vi "File Viewer v5.vi"() -> ()   [LabVIEW 2019]
uses:
  <vilib>/Utility/file.llb/Read Delimited Spreadsheet (I64).vi
  <vilib>/Utility/file.llb/Write Delimited Spreadsheet (DBL).vi
panel:
  in  "Stop":bool
  in  "Tab Control":T1(tab)
  in  "IR Filter:":u16(ring) items=["No filter", "100 nm Al", "200 nm Al", "250 nm Al", "500 nm Al"]
  in  "update":bool
  out "Raw Image From Camera":i32[][](graph)
  in  "File Path for Image:":path
  out "Expected position on spectrometer (pixels):":dbl
  in  "Grating:":u16(ring) items=["Shimadzu 30-006  "]
  in  "Laser:":u16(ring) items=["800nm  "]
  in  "Harmonic":dbl min=10.0 max=40.0
  out "l (nm)":dbl
  out "E (J)":dbl
  out "E (eV)":dbl
  out "Nearest Harmonic of 800nm":dbl
  out "Vertical Binned Waveform Graph":i64[](graph)
  out "Cursor Position (pixels)":dbl
  out "Distance to nearest harmonic of 800nm (pixels)":dbl
  in  "Caibration Date":u16(ring) items=["first calibration - 7/31", "7/31-current"]
  in  "Correct for QE?":bool
  in  "Save text file":bool
  in  "Graph to export:":u16(ring) items=["Wavelength Graph", "Energy Graph", "Harmonics Graph"]
  out "Wavelength Graph":T2(graph)
  out "Energy Graph (eV)":cluster{"eV":dbl, "QE scaled count":dbl}[](graph)
  out "Harmonics Graph":cluster{dbl, "QE scaled count":dbl}[](graph)
  in  "Pump/Probe Run Folder:":path
  out "Distance to nearest harmonic of 800nm (pixels)":dbl
  out "Cursor Position on CCD  (pixels)":dbl
  out "Nearest Harmonic of 800nm":dbl
  out "E (eV) 2":dbl
  out "E (J)":dbl
  out "l (nm)":dbl
  in  "Pump/Probe Harmonic:":dbl min=10.0 max=40.0
  out "Expected position on spectrometer (pixels):":dbl
  out "Time delay":dbl
  out "XUV":dbl[][](graph)
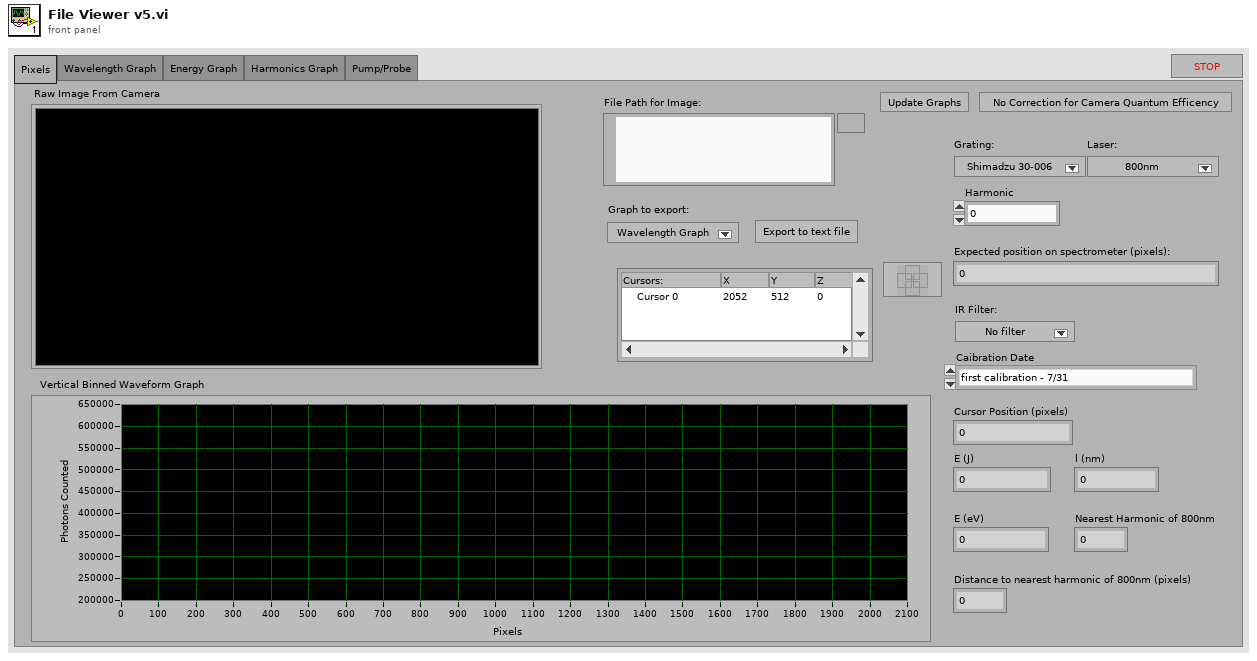
[diagram p1: front panel]
types:
  T1 = enum32{"Pixels", "Wavelength Graph", "Energy Graph", "Harmonics Graph", "Pump/Probe"}
  T2 = cluster{"No prefix":dbl, "QE scaled count":dbl}[]
  T3 = cluster{"No prefix":dbl, "filter scaled count":dbl}
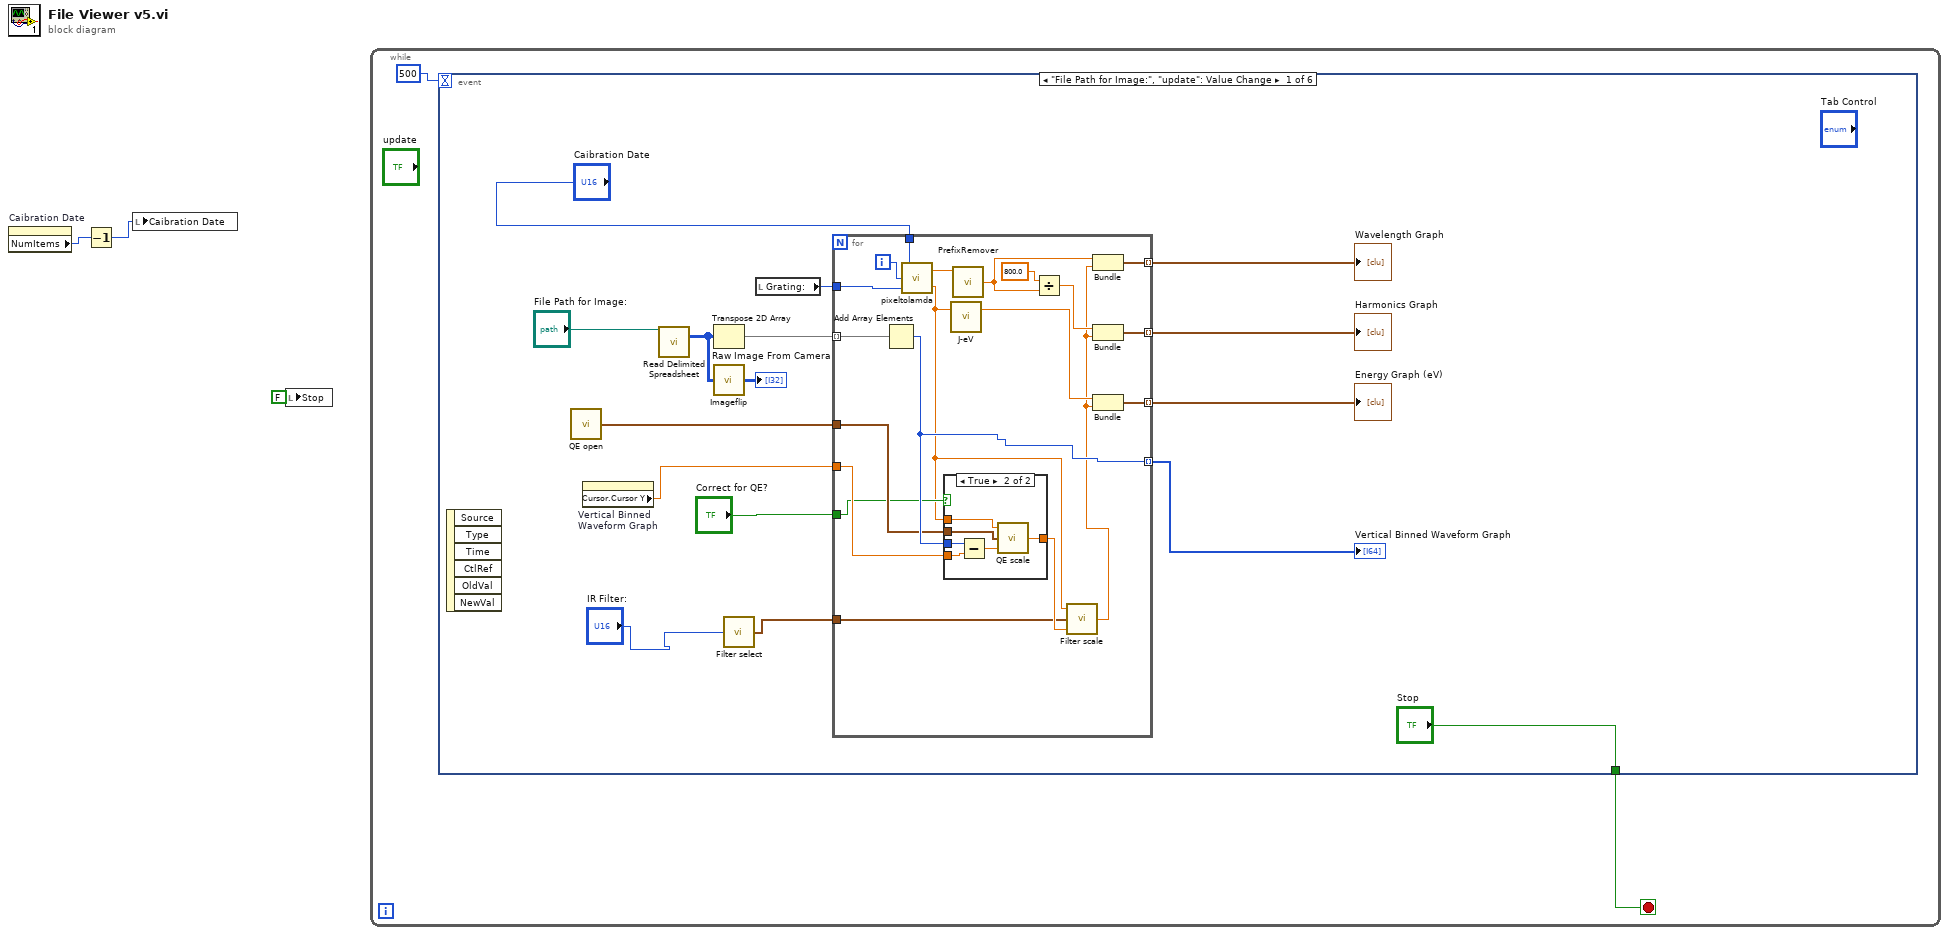
[diagram p0: block diagram]
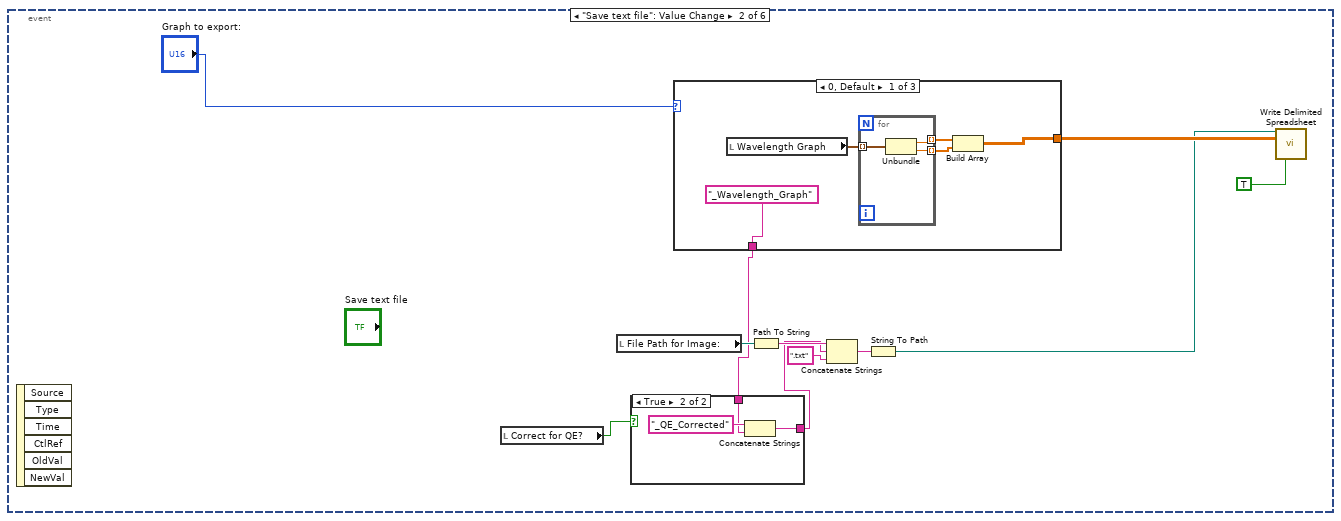
[diagram p3: hidden frame]
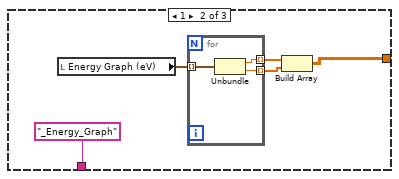
[diagram p5: hidden frame]
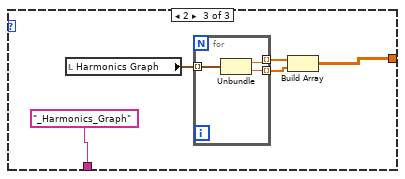
[diagram p6: hidden frame]
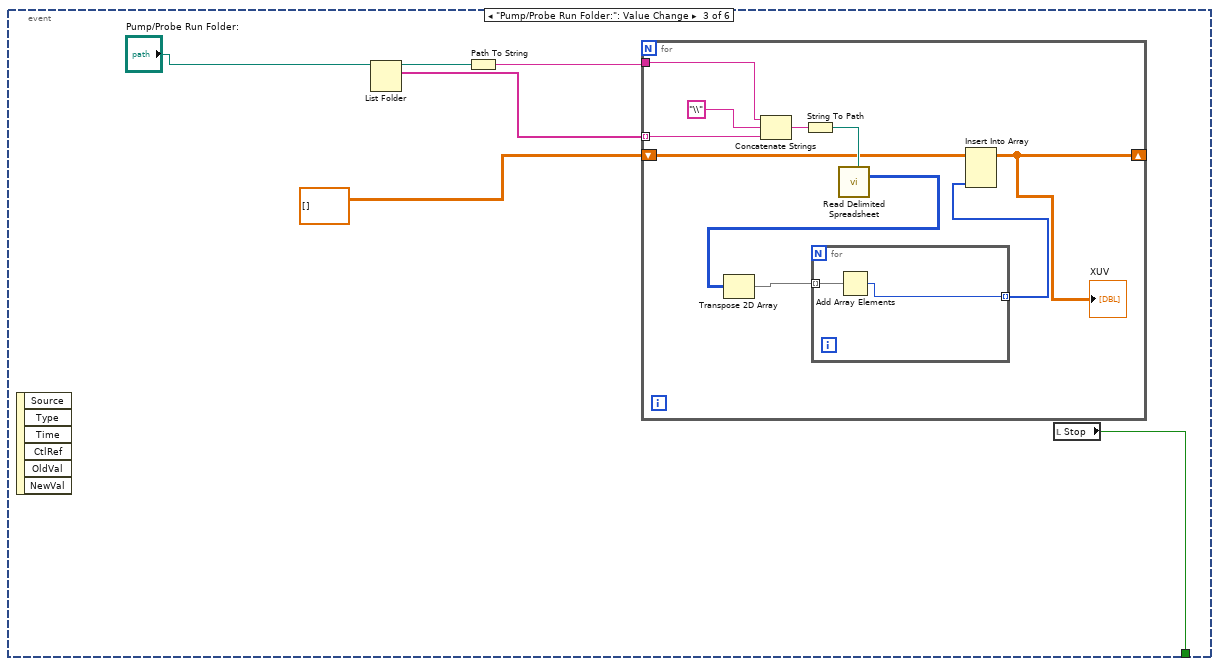
[diagram p7: hidden frame]
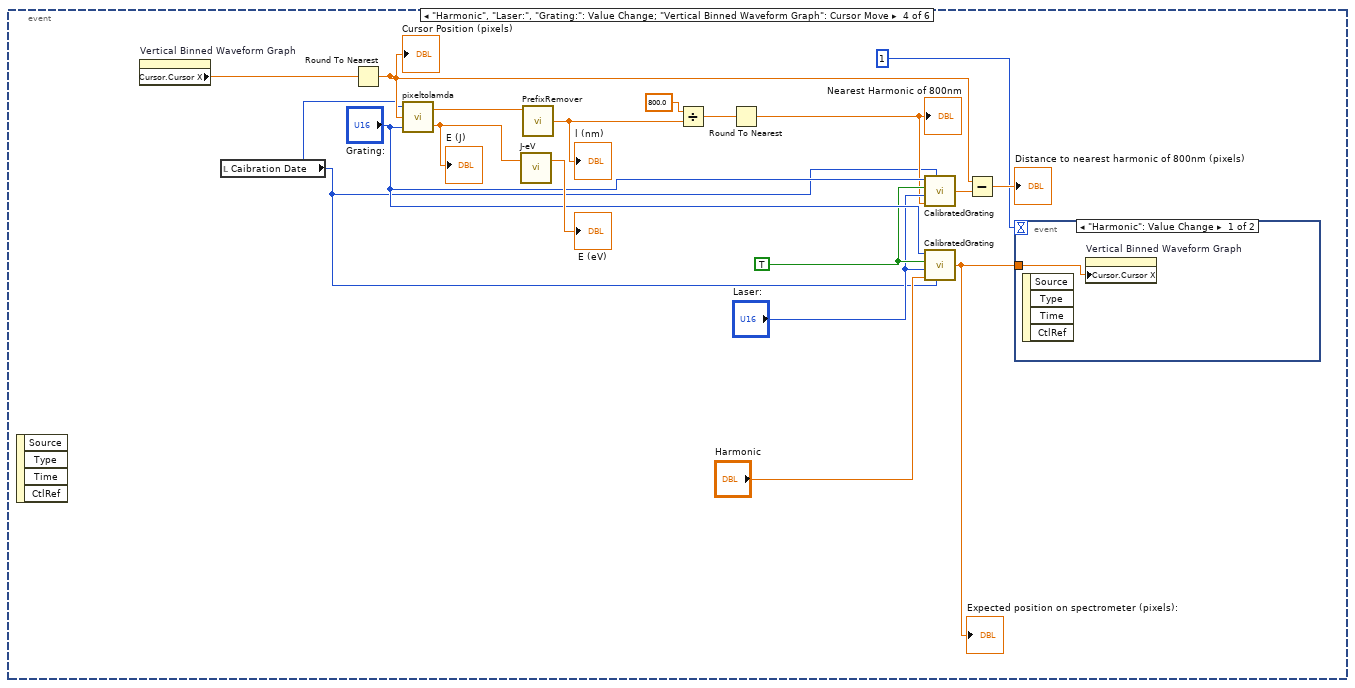
[diagram p8: hidden frame]
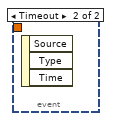
[diagram p9: hidden frame]
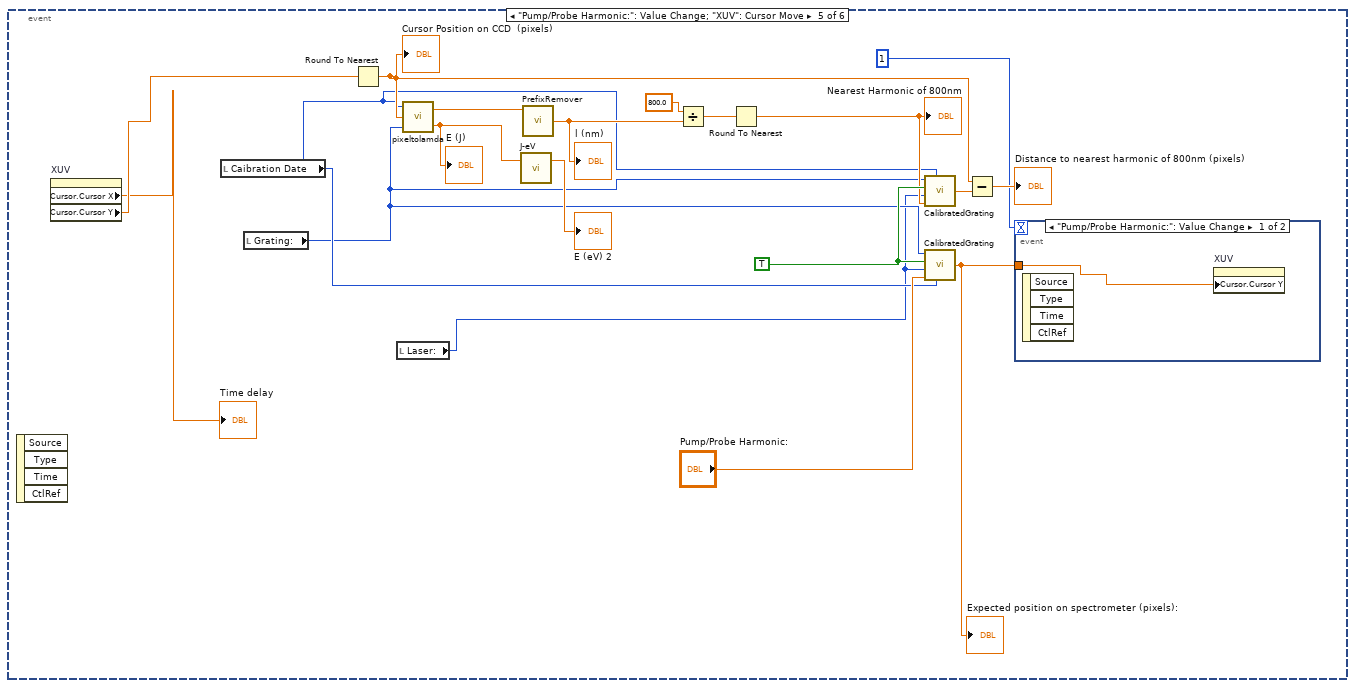
[diagram p10: hidden frame]
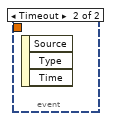
[diagram p11: hidden frame]
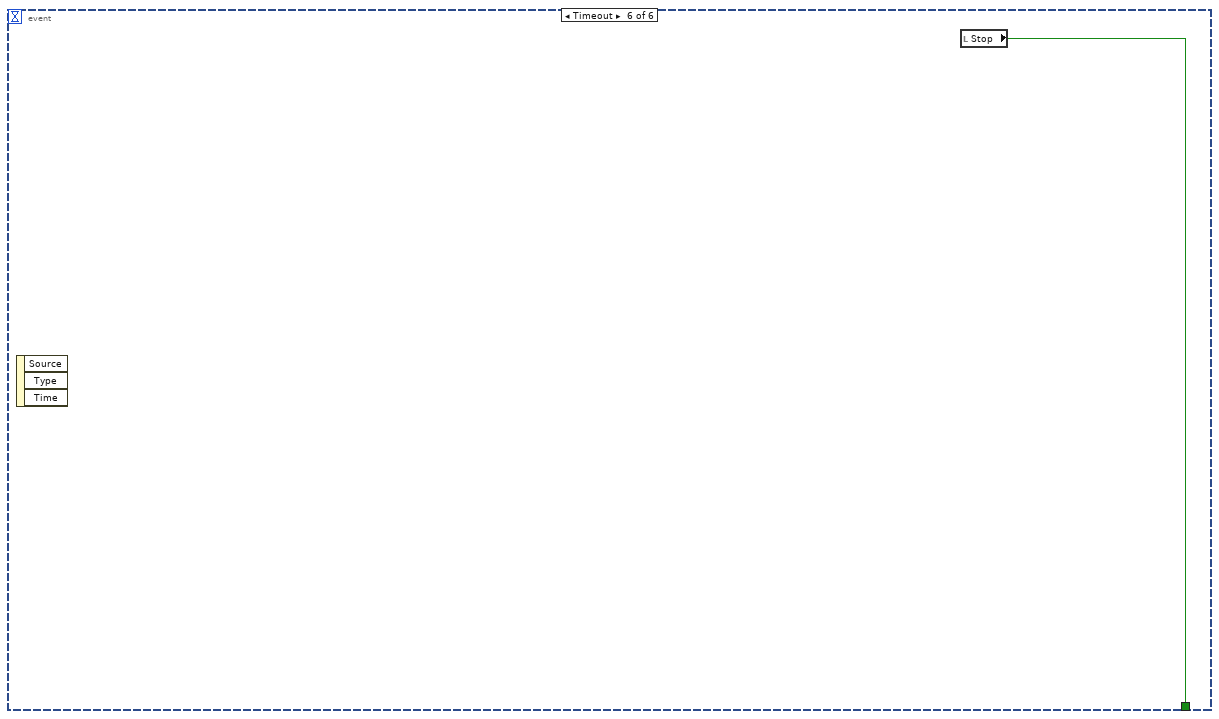
[diagram p12: hidden frame]
diagram:
  n1 = property on="Caibration Date" class="Ring (strict)"() -> ("NumItems"=w1:u32)  [unwired: 2 in, 2 out]
  n2 = Decrement(x=w1) -> (x-1=w2:u32)
  n3 = local write "Caibration Date"(w2) -> ()
  n4 = local write "Stop"(FALSE) -> ()
  n5 = while {
    stop <- w5 stop-if-true
    n6 = event shown="[0] \"File Path for Image:\", \"update\": Value Change" {
      selector: _ -> [_ _ _ _ _ _]
      dyn-events: _ -> [_ _ _ _ _ _]
      timeout: 500 -> [_ _ _ _ _ _]
      tunnel: ["Stop" _ w89 _ _ w145] -> w5
      event "File Path for Image:", "update": Value Change {
        n7 = event-data() -> ()  [unwired: 1 in, 6 out]
        n8 = call "QE open.vi"() -> ("QE data"=w10:cluster{"Numeric":dbl, dbl}[])
        n9 = property on="Vertical Binned Waveform Graph" class="WFGraph (strict)"() -> ("Cursor.Cursor Y"=w9:dbl)  [unwired: 2 in, 2 out]
        n10 = call-poly <vilib>:"Read Delimited Spreadsheet.vi"("file path (dialog if empty)"="File Path for Image:") -> ("all rows"=w18:i64[][])  [unwired: 9 in, 5 out]
        n11 = Transpose 2D Array(2D array=w18) -> (transposed array=w17:i64[][])
        n12 = call "Imageflip.vi"("2D array"=w18) -> ("transposed array"=→"Raw Image From Camera":i32[][])
        n13 = call "Filter select.vi"("Filter:"="IR Filter:") -> ("filter data"=w6:cluster{"Numeric":dbl, dbl}[])
        n14 = local read "Grating:"() -> (w15:u16)
        n15 = for {
          tunnel: w17 -> [w41] mode=indexing
          tunnel: [w29] -> w16 mode=indexing
          tunnel: w15 -> [w39]
          tunnel: [w38] -> w14 mode=indexing
          tunnel: [w37] -> w13 mode=indexing
          tunnel: [w32] -> w12 mode=indexing
          tunnel: "Caibration Date" -> [w31]
          tunnel: w10 -> [w28]
          tunnel: w9 -> [w30]
          tunnel: "Correct for QE?" -> [w26]
          tunnel: w6 -> [w22]
          i -> [w40]
          n16 = Add Array Elements(numeric array=w41) -> (sum=w29:i64)
          n17 = call "pixeltolamda.vi"("Grating:"=w39, "Pixel Postion"=w40, "Caibration Date"=w31) -> ("E (J)"=w23:dbl, "lamda (m)"=w35:dbl)
          n18 = case shown="True" w26 {
            tunnel: w30 -> [_ w48]
            tunnel: w29 -> [w42 w47]
            tunnel: w28 -> [_ w44]
            tunnel: w23 -> [_ w45]
            tunnel: [w42 w46] -> w25
            frame False {
            }
            frame True {
              n19 = Subtract(x=w47, y=w48) -> (x-y=w43:dbl)
              n20 = call "QE scale.vi"("Raw Photon Count"=w43, "QE data"=w44, "Energy (J)"=w45) -> ("QE scaled count"=w46:dbl)
            }
          }
          n21 = call "J-eV.vi"("J"=w23) -> ("eV"=w27:dbl)  [unwired: 1 in, 1 out]
          n22 = call "PrefixRemover.vi"("Nano"=w35) -> ("No prefix"=w34:dbl)  [unwired: 3 in]
          n23 = Divide(x=800.0, y=w34) -> (x/y=w33:dbl)
          n24 = call "Filter scale.vi"("Raw Photon Count"=w25, "filter data"=w22, "Energy (J)"=w23) -> ("filter scaled count"=w24:dbl)
          n25 = Bundle("No prefix"=w34, "filter scaled count"=w24) -> (w38:T3)  [unwired: 1 in]
          n26 = Bundle(w33, "filter scaled count"=w24) -> (w32:cluster{dbl, "filter scaled count":dbl})  [unwired: 1 in]
          n27 = Bundle("eV"=w27, "filter scaled count"=w24) -> (w37:cluster{"eV":dbl, "filter scaled count":dbl})  [unwired: 1 in]
        }
        "Vertical Binned Waveform Graph" <- w16
        "Wavelength Graph" <- w14
        "Energy Graph (eV)" <- w13
        "Harmonics Graph" <- w12
      }
      event "Save text file": Value Change {
        n28 = event-data() -> ()  [unwired: 1 in, 6 out]
        n29 = local read "Correct for QE?"() -> (w53:bool)
        n30 = local read "File Path for Image:"() -> (w56:path)
        n31 = case shown="0, Default" "Graph to export:" {
          tunnel: [w65 w73 w81] -> w58
          tunnel: ["_Wavelength_Graph" ("pattern (all files)") "_Energy_Graph" ("pattern (all files)") "_Harmonics_Graph" ("pattern (all files)")] -> w51
          frame 0, Default {
            n32 = local read "Wavelength Graph"() -> (w68:T2)
            n33 = for {
              tunnel: w68 -> [w71] mode=indexing
              tunnel: [w70] -> w67 mode=indexing
              tunnel: [w69] -> w66 mode=indexing
              n34 = Unbundle(w71) -> ("No prefix"=w70:dbl, "QE scaled count"=w69:dbl)
            }
            n35 = Build Array(w67, w66) -> (w65:dbl[][])
          }
          frame 1 {
            n36 = local read "Energy Graph (eV)"() -> (w74:cluster{"eV":dbl, "QE scaled count":dbl}[])
            n37 = for {
              tunnel: w74 -> [w79] mode=indexing
              tunnel: [w78] -> w76 mode=indexing
              tunnel: [w77] -> w75 mode=indexing
              n38 = Unbundle(w79) -> ("eV"=w78:dbl, "QE scaled count"=w77:dbl)
            }
            n39 = Build Array(w76, w75) -> (w73:dbl[][])
          }
          frame 2 {
            n40 = local read "Harmonics Graph"() -> (w82:cluster{dbl, "QE scaled count":dbl}[])
            n41 = for {
              tunnel: w82 -> [w87] mode=indexing
              tunnel: [w86] -> w84 mode=indexing
              tunnel: [w85] -> w83 mode=indexing
              n42 = Unbundle(w87) -> (w86:dbl, "QE scaled count"=w85:dbl)
            }
            n43 = Build Array(w84, w83) -> (w81:dbl[][])
          }
        }
        n44 = case shown="True" w53 {
          tunnel: [w60 w62] -> w52
          tunnel: w51 -> [w60 w61]
          frame False {
          }
          frame True {
            n45 = Concatenate Strings("_QE_Corrected" ("pattern (all files)"), w61) -> (w62:string)
          }
        }
        n46 = Path To String(path=w56) -> (string=w55:string)
        n47 = Concatenate Strings(w55, w52, ".txt" ("pattern (all files)")) -> (w50:string)
        n48 = String To Path(string=w50) -> (path=w49:path)
        n49 = call-poly <vilib>:"Write Delimited Spreadsheet.vi"("file path (dialog if empty)"=w49, "2D data"=w58, "transpose? (no:F)"=TRUE) -> ()  [unwired: 11 in, 2 out]
      }
      event "Pump/Probe Run Folder:": Value Change {
        n50 = event-data() -> ()  [unwired: 1 in, 6 out]
        n51 = List Folder(path="Pump/Probe Run Folder:") -> (path out=w91:path, filenames=w92:string[])  [unwired: 3 in, 2 out]
        n52 = Path To String(path=w91) -> (string=w90:string)
        n53 = for {
          tunnel: w92 -> [w101] mode=indexing
          tunnel: w90 -> [w99]
          shift-right: [w94] -> _
          shift-left: dbl[][] [] -> [w98]
          n54 = Concatenate Strings(w99, "\\" ("string"), w101) -> (w103:string)
          n55 = String To Path(string=w103) -> (path=w102:path)
          n56 = call-poly <vilib>:"Read Delimited Spreadsheet.vi"("file path (dialog if empty)"=w102) -> ("all rows"=w96:i64[][])  [unwired: 9 in, 5 out]
          n57 = Transpose 2D Array(2D array=w96) -> (transposed array=w95:i64[][])
          n58 = for {
            tunnel: w95 -> [w105] mode=indexing
            tunnel: [w104] -> w97 mode=indexing
            n59 = Add Array Elements(numeric array=w105) -> (sum=w104:i64)
          }
          n60 = Insert Into Array(array=w98, new element=w97) -> (w94:dbl[][])  [unwired: 2 in]
          "XUV" <- w94
        }
        n61 = local read "Stop"() -> (w89:bool)
      }
      event "Harmonic", "Laser:", "Grating:": Value Change; "Vertical Binned Waveform Graph": Cursor Move {
        w115 = TRUE ("Subvi?")
        n62 = event-data() -> ()  [unwired: 1 in, 4 out]
        n63 = property on="Vertical Binned Waveform Graph" class="WFGraph (strict)"() -> ("Cursor.Cursor X"=w117:dbl)  [unwired: 2 in, 2 out]
        n64 = local read "Caibration Date"() -> (w106:u16)
        n65 = Round To Nearest(number=w117) -> (nearest integer value=w109:dbl)
        "Cursor Position (pixels)" <- w109
        n66 = call "pixeltolamda.vi"("Grating:"="Grating:", "Pixel Postion"=w109, "Caibration Date"=w106) -> ("E (J)"=w121:dbl, "lamda (m)"=w122:dbl)
        "E (J)" <- w121
        n67 = call "J-eV.vi"("J"=w121) -> ("eV"=→"E (eV)":dbl)  [unwired: 1 in, 1 out]
        n68 = call "PrefixRemover.vi"("Nano"=w122) -> ("No prefix"=w112:dbl)  [unwired: 3 in]
        "l (nm)" <- w112
        n69 = Divide(x=800.0, y=w112) -> (x/y=w119:dbl)
        n70 = Round To Nearest(number=w119) -> (nearest integer value=w113:dbl)
        "Nearest Harmonic of 800nm" <- w113
        n71 = call "CalibratedGrating.vi"("Grating:"="Grating:", "Subvi?"=w115, "Laser:"="Laser:", "Harmonic"=w113, "Caibration Date"=w106) -> ("Position on spectrometer (pixels):"=w111:dbl)
        n72 = call "CalibratedGrating.vi"("Grating:"="Grating:", "Subvi?"=w115, "Laser:"="Laser:", "Harmonic"="Harmonic", "Caibration Date"=w106) -> ("Position on spectrometer (pixels):"=w108:dbl)
        "Expected position on spectrometer (pixels):" <- w108
        n73 = Subtract(x=w109, y=w111) -> (x-y=→"Distance to nearest harmonic of 800nm (pixels)":dbl)
        n74 = event shown="[0] \"Harmonic\": Value Change" {
          selector: _ -> [_ _]
          dyn-events: _ -> [_ _]
          timeout: 1 -> [_ _]
          tunnel: w108 -> [w124 _]
          event "Harmonic": Value Change {
            n75 = event-data() -> ()  [unwired: 1 in, 4 out]
            n76 = property on="Vertical Binned Waveform Graph" class="WFGraph (strict)"("Cursor.Cursor X"=w124) -> ()  [unwired: 2 in, 2 out]
          }
          event Timeout {
            n77 = event-data() -> ()  [unwired: 1 in, 3 out]
          }
        }
      }
      event "Pump/Probe Harmonic:": Value Change; "XUV": Cursor Move {
        w137 = TRUE ("Subvi?")
        n78 = event-data() -> ()  [unwired: 1 in, 4 out]
        n79 = property on="XUV" class="IntGraph (strict)"() -> ("Cursor.Cursor X"=→"Time delay":dbl, "Cursor.Cursor Y"=w126:dbl)  [unwired: 2 in, 2 out]
        n80 = local read "Caibration Date"() -> (w129:u16)
        n81 = local read "Grating:"() -> (w128:u16)
        n82 = Round To Nearest(number=w126) -> (nearest integer value=w132:dbl)
        "Cursor Position on CCD  (pixels)" <- w132
        n83 = local read "Laser:"() -> (w127:u16)
        n84 = call "pixeltolamda.vi"("Grating:"=w128, "Pixel Postion"=w132, "Caibration Date"=w129) -> ("E (J)"=w141:dbl, "lamda (m)"=w142:dbl)
        "E (J)" <- w141
        n85 = call "J-eV.vi"("J"=w141) -> ("eV"=→"E (eV) 2":dbl)  [unwired: 1 in, 1 out]
        n86 = call "PrefixRemover.vi"("Nano"=w142) -> ("No prefix"=w135:dbl)  [unwired: 3 in]
        "l (nm)" <- w135
        n87 = Divide(x=800.0, y=w135) -> (x/y=w139:dbl)
        n88 = Round To Nearest(number=w139) -> (nearest integer value=w136:dbl)
        "Nearest Harmonic of 800nm" <- w136
        n89 = call "CalibratedGrating.vi"("Grating:"=w128, "Subvi?"=w137, "Laser:"=w127, "Harmonic"=w136, "Caibration Date"=w129) -> ("Position on spectrometer (pixels):"=w134:dbl)
        n90 = call "CalibratedGrating.vi"("Grating:"=w128, "Subvi?"=w137, "Laser:"=w127, "Harmonic"="Pump/Probe Harmonic:", "Caibration Date"=w129) -> ("Position on spectrometer (pixels):"=w131:dbl)
        "Expected position on spectrometer (pixels):" <- w131
        n91 = Subtract(x=w132, y=w134) -> (x-y=→"Distance to nearest harmonic of 800nm (pixels)":dbl)
        n92 = event shown="[0] \"Pump/Probe Harmonic:\": Value Change" {
          selector: _ -> [_ _]
          dyn-events: _ -> [_ _]
          timeout: 1 -> [_ _]
          tunnel: w131 -> [w144 _]
          event "Pump/Probe Harmonic:": Value Change {
            n93 = event-data() -> ()  [unwired: 1 in, 4 out]
            n94 = property on="XUV" class="IntGraph (strict)"("Cursor.Cursor Y"=w144) -> ()  [unwired: 2 in, 2 out]
          }
          event Timeout {
            n95 = event-data() -> ()  [unwired: 1 in, 3 out]
          }
        }
      }
      event Timeout {
        n96 = event-data() -> ()  [unwired: 1 in, 3 out]
        n97 = local read "Stop"() -> (w145:bool)
      }
    }
  }
